vi "Timer Interrupt Handling.vi"() -> ()   [LabVIEW 2021]
uses:
  <vilib>/myRIO/Express VI/IRQ/IRQ Express VI.xnode
  <vilib>/myRIO/Instrument Drivers/Utilities/Utilities.lvlib
  <vilib>/myRIO/Express VI/Onboard Devices/LED/LED Express VI.xnode
  <vilib>/myRIO/Common/Instrument Driver Framework/myRIO v1.0/IRQ/typedefs/Callback VI Ref.ctl
  <vilib>/myRIO/Instrument Drivers/IRQ/Timer IRQ/vis/myRIO Create Timer IRQ.xnode
  <vilib>/myRIO/Common/Instrument Driver Framework/myRIO v1.0/IRQ/vis/myRIO v1.1 Create Timer IRQ.vi
  <vilib>/userdefined/High Color/nirio_resource_hc.ctl
  Timer Callback 1CPU.vi
  Timer Callback 2CPUs.vi
  <vilib>/myRIO/Instrument Drivers/Onboard IO/DIO/vis/Write.vi
  <vilib>/myRIO/Instrument Drivers/Onboard IO/DIO/DIO.lvlib
  <vilib>/myRIO/Common/Instrument Driver Framework/myRIO v1.0/DIO/typedefs/DIO Channels Enum.ctl
  <vilib>/myRIO/Common/Instrument Driver Framework/myRIO v1.0/DIO/typedefs/DIO Channels List.ctl
  <vilib>/myRIO/Common/Instrument Driver Framework/Utilities/typedefs/Generic FPGA Reference.ctl
  <vilib>/myRIO/Common/Instrument Driver Framework/Utilities/typedefs/myRIO v1.0 Reference.ctl
  <vilib>/myRIO/Common/Instrument Driver Framework/Utilities/typedefs/Hardware Version Enum.ctl
  <vilib>/myRIO/Common/Instrument Driver Framework/Utilities/typedefs/myRIO Generic Hardware Reference.ctl
  <vilib>/myRIO/Instrument Drivers/Onboard IO/DIO/typedefs/DIO Reference.ctl
  <vilib>/myRIO/Instrument Drivers/Onboard IO/DIO/vis/myRIO DIO Open.xnode
  <vilib>/myRIO/Common/Instrument Driver Framework/Utilities/vis/Is FPGA Ref Available.vi
  <vilib>/myRIO/Common/Instrument Driver Framework/myRIO v1.0/DIO/vis/myRIO v1.1 Open DIO.vi
panel:
  in  "Mode":T1(ring)
  out "error out":errorcluster
  in  "stop":bool
  # "Overview: This VI demonstrates how to use callback VIs to handle a timer interrupt.\nInstructions:\n1.\tIn the Project Explorer window, verify the IP address of the myRIO target. If it is incorrect, update the IP address.\n2.\tRun the VI.\n3.\tObserve the LEDs on the myRIO. The LEDs continuously light up in sequence.\n4.\tThe VI triggers an interrupt every 5 seconds. When an interrupt occurs, observe the changes of the way how the LEDs light up.\n5.\tThe VI includes two callback VIs. One VI uses one CPU, whereas the other VI uses two CPUs. To see the different impacts between the two modes, change the value of Mode."
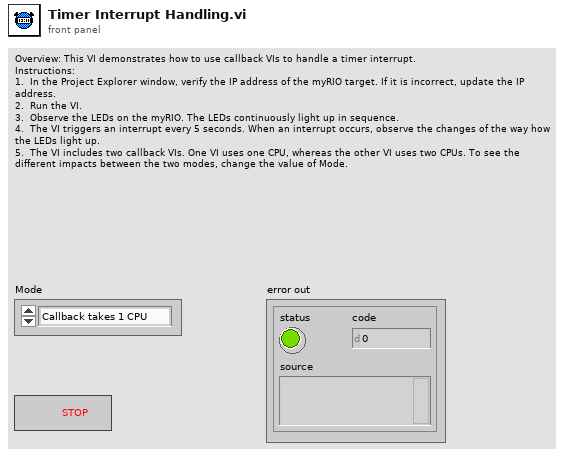
[diagram p1: front panel]
types:
  T1 = enum16{"Callback takes 1 CPU", "Callback takes 2 CPUs"}
  T2 = typedef "nirio_resource_hc.ctl" = tag
  T3 = typedef "DIO.lvlib/DIO Reference.ctl" = cluster{"myRIO Reference":T4, "DIO Channels List":T8}
  T4 = typedef "myRIO Generic Hardware Reference.ctl" = cluster{"myRIO Model":T5, "myRIO Hardware Reference":T6}
  T5 = typedef "Hardware Version Enum.ctl" = enum16{"Unknown", "myRIO-1900", "myRIO-1950", "roboRIO", "NI ELVIS RIO CM", "ELVIS III"}
  T6 = typedef "myRIO v1.0 Reference.ctl" = cluster{"Generic FPGA Reference":T7, "Allow multiple opens":bool}
  T7 = typedef "Generic FPGA Reference.ctl" = refnum<k20>
  T8 = typedef "DIO Channels List.ctl" = T9[]
  T9 = typedef "DIO Channels Enum.ctl" = enum16{"Not Connected", "C/DIO0", "C/DIO1", "C/DIO2", "C/DIO3", "C/DIO4", "C/DIO5", "C/DIO6", "C/DIO7", "A/DIO0", "A/DIO1", "A/DIO2", "A/DIO3", "A/DIO4", "A/DIO5", "A/DIO6", "A/DIO7", "A/DIO8", "A/DIO9", "A/DIO10", "A/DIO11", "A/DIO12", "A/DIO13", "A/DIO14", "A/DIO15", "A/DIO16", "A/DIO17", "A/DIO18", "A/DIO19", "B/DIO0", "B/DIO1", "B/DIO2", "B/DIO3", "B/DIO4", "B/DIO5", "B/DIO6", "B/DIO7", "B/DIO8", "B/DIO9", "B/DIO10", "B/DIO11", "B/DIO12", "B/DIO13", "B/DIO14", "B/DIO15", "B/DIO16", "B/DIO17", "B/DIO18", "B/DIO19", "LED0", "LED1", "LED2", "LED3", "Button0", "DIO/DIO0", "DIO/DIO1", "DIO/DIO2", "DIO/DIO3", "DIO/DIO4", "DIO/DIO5", "DIO/DIO6", "DIO/DIO7", "DIO/DIO8", "DIO/DIO9", "SPI/CS0", "SPI/CS1", "SPI/CS2", "SPI/CS3", "LED RADIO (Green)", "LED RADIO (Red)", "LED COMM (Green)", "LED COMM (Red)", "LED MODE (Green)", "LED MODE (Red)"}
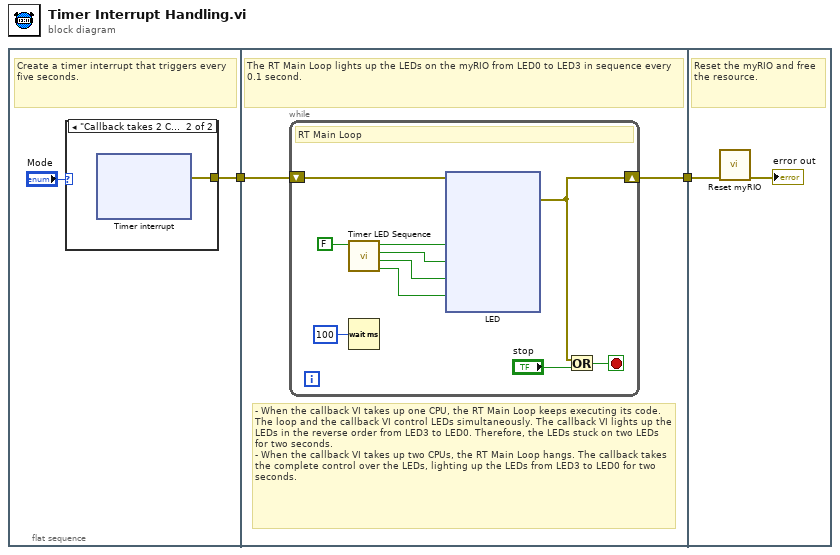
[diagram p0: block diagram]
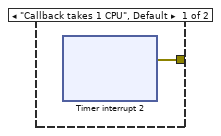
[diagram p2: hidden frame]
diagram:
  n1 = flat-sequence {
    tunnel: [w4] -> w1
    tunnel: [w33] -> w2
    tunnel: w1 -> [w34]
    tunnel: w2 -> [w84]
    frame #0 {
      # "Create a timer interrupt that triggers every five seconds."
      n2 = case shown="\"Callback takes 2 CPUs\"" "Mode" {
        tunnel: [w5 w19] -> w4
        frame "Callback takes 1 CPU", Default {
          n3 = xnode "Timer interrupt 2"() -> ("error out"=w5:errorcluster)  [unwired: 1 in]
        }
        frame "Callback takes 2 CPUs" {
          n4 = xnode "Timer interrupt"() -> ("error out"=w19:errorcluster)  [unwired: 1 in]
        }
      }
    }
    frame #1 {
      # "- When the callback VI takes up one CPU, the RT Main Loop keeps executing its code. The loop and the callback VI control LEDs simultaneously. The callback VI lights up the LEDs in the reverse order from LED3 to LED0. Therefore, the LEDs stuck on two LEDs for two seconds.\n- When the callback VI takes up two CPUs, the RT Main Loop hangs. The callback takes the complete control over the LEDs, lighting up the LEDs from LED3 to LED0 for two seconds."
      # "The RT Main Loop lights up the LEDs on the myRIO from LED0 to LED3 in sequence every 0.1 second."
      n5 = while {
        shift-right: [w41] -> w33
        shift-left: w34 -> [w40]
        stop <- w42 stop-if-true
        # "RT Main Loop"
        n6 = call "Timer LED Sequence.vi"("Reverse?"=FALSE) -> ("LED3"=w36:bool, "LED2"=w37:bool, "LED1"=w38:bool, "LED0"=w39:bool)  [unwired: 7 in]
        n7 = Wait (ms)(milliseconds to wait=u32 100) -> ()  [unwired: 1 out]
        n8 = xnode "LED"("LED0"=w39, "LED1"=w38, "LED2"=w37, "LED3"=w36, "error in (no error)"=w40) -> ("error out"=w41:errorcluster)
        n9 = Or(x=w41, y="stop") -> (x .or. y?=w42:bool)
      }
    }
    frame #2 {
      # "Reset the myRIO and free the resource."
      n10 = call <vilib>:"Reset myRIO.vi"("error in (no error)"=w84) -> ("error out"=→"error out":errorcluster)  [unwired: 10 in]
    }
  }
